vi "PDash - Rename DQMH Event.vi"(9 "New Event Name":string, 10 "Event Info (Existing)":T1={"Event VI Path"=path "", "Argument Path"=path "", "Wait Argument Path"=path "", "Event Arg Owner"=-1, "Event Name"="", "Type"=enum."Request"}, 11 "Module Info":T3) -> (0 "error out":errorcluster)   [LabVIEW 2019]
doc: "_____\nCreated using DQMH Event Scripter 7.1.0.1447."
uses:
  <vilib>/Delacor/Delacor QMH/Libraries/_Scripting Support/Module Info--cluster.ctl
  <vilib>/Delacor/Delacor QMH/Libraries/_Scripting Support/Module Type--enum.ctl
  <vilib>/Delacor/Delacor QMH/Libraries/_Scripting Support/Event Info (Existing)--cluster.ctl
  Program Files (x86)/National Instruments/LabVIEW 2019/project/Delacor/DQMH/_DQMH Remove Event/Event Type (All Permutations)--enum.ctl
  PantherDashboard Scripting Hooks/Panther Dasboard Scripting Hooks.lvlib
  <vilib>/Delacor/Delacor QMH/Libraries/_Scripting Support/dqmh_lib_DQMH Scripting Support.lvlib
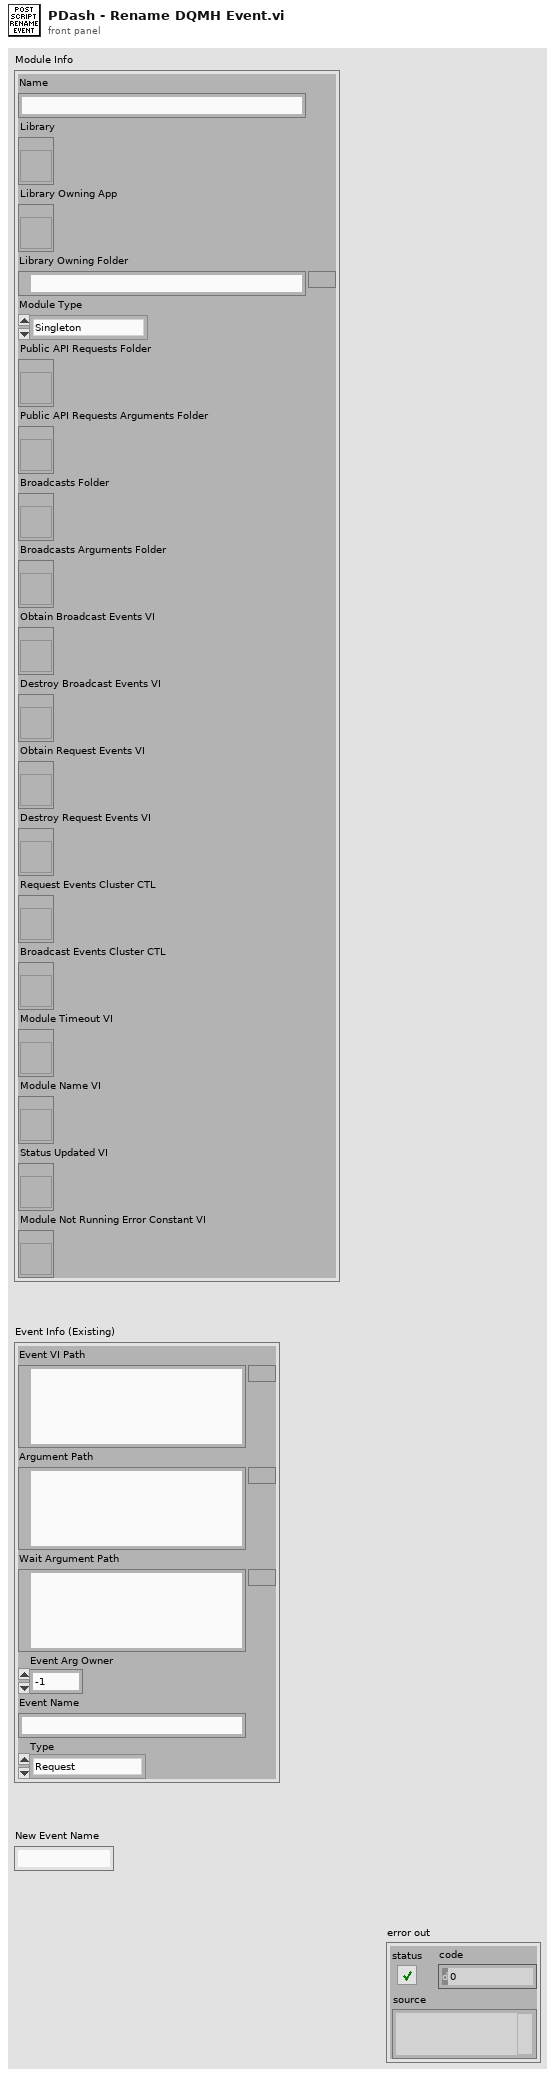
[diagram p1: front panel]
types:
  T1 = typedef "dqmh_lib_DQMH Scripting Support.lvlib/Event Info (Existing)--cluster.ctl" = cluster{"Event VI Path":path, "Argument Path":path, "Wait Argument Path":path, "Event Arg Owner":i32, "Event Name":string, "Type":T2}
  T2 = typedef "dqmh_lib_DQMH Scripting Support.lvlib/Event Type (All Permutations)--enum.ctl" = enum16{"Request", "Broadcast", "Both", "Request (no Wait)", "Request and Wait", "Request (Private)", "Request (Local Instance)"}
  T3 = typedef "dqmh_lib_DQMH Scripting Support.lvlib/Module Info--cluster.ctl" = cluster{"Name":string, "Library":refnum<vi>, "Library Owning App":refnum<vi>, "Library Owning Folder":path, "Module Type":T4, "Public API Requests Folder":refnum<vi>, "Public API Requests Arguments Folder":refnum<vi>, "Broadcasts Folder":refnum<vi>, "Broadcasts Arguments Folder":refnum<vi>, "Obtain Broadcast Events VI":refnum<vi>, "Destroy Broadcast Events VI":refnum<vi>, "Obtain Request Events VI":refnum<vi>, "Destroy Request Events VI":refnum<vi>, "Request Events Cluster CTL":refnum<vi>, "Broadcast Events Cluster CTL":refnum<vi>, "Module Timeout VI":refnum<vi>, "Module Name VI":refnum<vi>, "Status Updated VI":refnum<vi>, "Module Not Running Error Constant VI":refnum<vi>}
  T4 = typedef "dqmh_lib_DQMH Scripting Support.lvlib/Module Type--enum.ctl" = enum16{"Singleton", "Cloneable"}
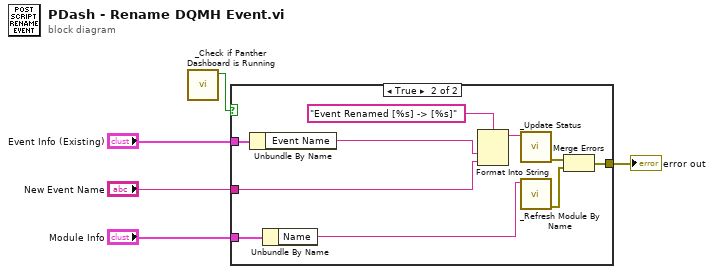
[diagram p0: block diagram]
diagram:
  n1 = call "_Check if Panther Dashboard is Running.vi"() -> ("Panther Dashboard is Running?"=w3:bool)  [unwired: 10 in, 1 out]
  n2 = case shown="True" w3 {
    tunnel: "Module Info" -> [_ w12]
    tunnel: [_ w14] -> w5
    tunnel: "New Event Name" -> [_ w10]
    tunnel: "Event Info (Existing)" -> [_ w9]
    frame False {
    }
    frame True {
      n3 = Unbundle By Name(w9) -> ("Event Name"=w8:string)
      n4 = Unbundle By Name(w12) -> ("Name"=w11:string)
      n5 = Format Into String(format string="Event Renamed [%s] -> [%s]", w8, w10) -> (resulting string=w7:string)  [unwired: 2 in, 1 out]
      n6 = call "_Update Status.vi"("Status"=w7) -> ("error out"=w13:errorcluster)  [unwired: 10 in]
      n7 = call "_Refresh Module By Name.vi"("Module Name"=w11) -> ("error out"=w15:errorcluster)  [unwired: 10 in]
      n8 = Merge Errors(w13, w15) -> (w14:errorcluster)
    }
  }
  "error out" <- w5
